vi "Diagnostic Global (U32).vi"() -> ()   [LabVIEW 2019]
panel:
  in  "Diag Global (U32)":u32[](array[numeric])=[0, 0, 0, 0, 0, 0]
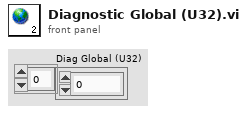
[diagram p1: front panel]
diagram:
